vi "Run.vi"(7 "Team Index":i32, 8 "Column":i32, 9 "Row":i32, 10 "View":i32[](array[numeric]) caption="View (Team Index, -1: empty)", 11 "Team 3 In":refnum<class "Team 3.lvclass">) -> (0 "Replicated":refnum<class "Square.lvclass">, 1 "Direction":T1, 2 "Action":T2, 3 "Square Out":refnum<class "Square.lvclass">)   [LabVIEW 2020, in "Team 3.lvclass"]
uses:
  Team 3.lvclass
  C:/dev/IlluminatedG/sol-squarebattle/Square/Square.lvclass
  Square/Square.lvclass
  Type Defs/Action Enum.ctl
  Type Defs/Direction Enum.ctl
  Team 3.lvclass/Team 3.ctl
  SubVIs/Read-Only Globals.vi
  SubVIs/Globals (private).vi
  SubVIs/Read-Only Stats.vi
  DS Square Library/DS Square.lvlib
  Type Defs/SB Type Defs.lvlib
panel:
  # "NW\nN\nNE\nE\nSE\nS\nSW\nW"
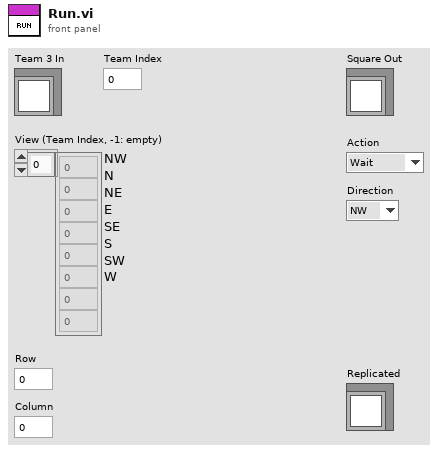
[diagram p1: front panel]
types:
  T1 = typedef "SB Type Defs.lvlib/Direction Enum.ctl" = enum16{"NW", "N", "NE", "E", "SE", "S", "SW", "W"}
  T2 = typedef "SB Type Defs.lvlib/Action Enum.ctl" = enum16{"Wait", "Move", "Attack", "Replicate"}
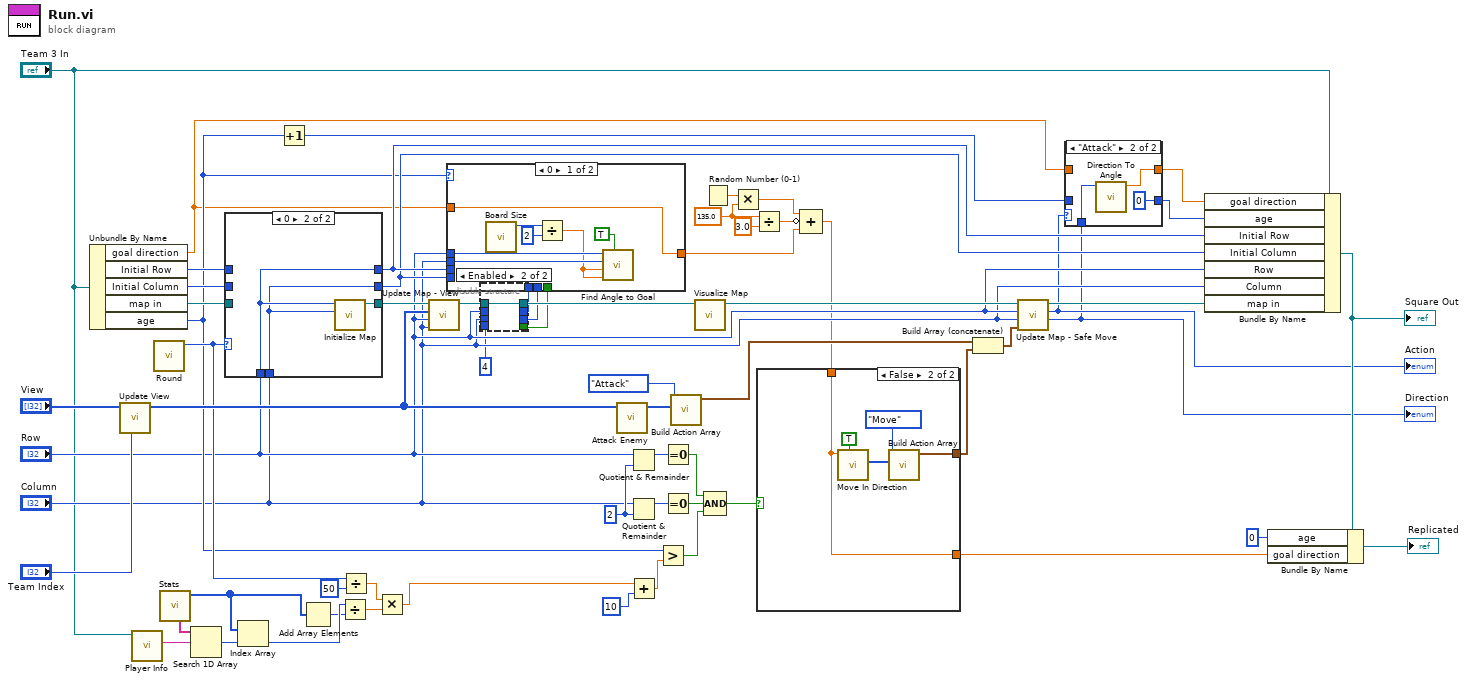
[diagram p0: block diagram]
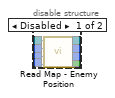
[diagram p3: hidden frame]
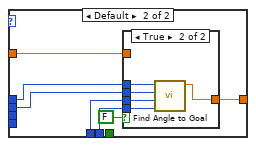
[diagram p4: hidden frame]
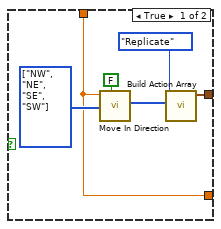
[diagram p6: hidden frame]
diagram:
  w41 = 135.0 ("y")
  w59 = 2 ("y")
  n1 = Unbundle By Name("Team 3 In") -> ("goal direction"=w1:dbl, "Initial Row"=w38:i32, "Initial Column"=w37:i32, "map in"=w63:refnum<data-value>, "age"=w28:i32)
  n2 = call "Update View.vi"("Team Index"="Team Index", "View"="View") -> ("View out"=w53:i32[])  [unwired: 9 in]
  n3 = call-dynamic "Player Info.vi"("Team 3 in"="Team 3 In") -> ("Name"=w17:string)  [unwired: 7 in, 3 out]
  n4 = call "Round.vi"() -> ("Round"=w31:i32)  [unwired: 11 in]
  n5 = call "Stats.vi"() -> ("Squares"=w16:i32[], "Players"=w18:string[])  [unwired: 7 in, 3 out]
  n6 = Search 1D Array(1D array=w18, element=w17) -> (index of element=w15:i32)  [unwired: 1 in]
  n7 = case shown="0" w31 {
    tunnel: w63 -> [w66 _]
    tunnel: [w66 w69] -> w62
    tunnel: "Column" -> [_ w67]
    tunnel: "Row" -> [_ w68]
    tunnel: w38 -> [w65 _]
    tunnel: w37 -> [w64 _]
    tunnel: [w65 w68] -> w36
    tunnel: [w64 w67] -> w35
    frame Default {
    }
    frame 0 {
      n8 = call "Initialize Map.vi"("Column"=w67, "Row"=w68) -> ("map"=w69:refnum<data-value>)  [unwired: 9 in]
    }
  }
  n9 = Index Array(array=w16, index=w15) -> (element=w14:i32)
  n10 = Increment(x=w28) -> (x+1=w4:i32)
  n11 = Add Array Elements(numeric array=w16) -> (sum=w13:i32)
  n12 = Divide(x=w14, y=w13) -> (x/y=w11:dbl)
  n13 = Divide(x=w31, y=50) -> (x/y=w12:dbl)
  n14 = Multiply(x=w12, y=w11) -> (x*y=w10:dbl)
  n15 = call "Update Map - View.vi"("Column"="Column", "Row"="Row", "Updated View"=w53, "map in"=w62) -> ("map out"=w27:refnum<data-value>)  [unwired: 7 in]
  n16 = disable-structure shown="Enabled" {
    disable-tunnel: w27 -> [w77 w78]
    disable-tunnel: [w76 w78] -> w26
    disable-tunnel: "Row" -> [w75 _]
    disable-tunnel: "Column" -> [w74 _]
    disable-tunnel: [w73 _] -> w23
    disable-tunnel: [w72 _] -> w22
    disable-tunnel: [w71 _] -> w21
    disable-tunnel: 4 ("distance (10)") -> [w70 _]
    frame Disabled {
      n17 = call "Read Map - Enemy Position.vi"("distance (10)"=w70, "column"=w74, "row"=w75, "map in"=w77) -> ("found?"=w73:bool, "enemy column"=w72:i32, "enemy row"=w71:i32, "map out"=w76:refnum<data-value>)  [unwired: 3 in, 1 out]
    }
    frame Enabled {
    }
  }
  n18 = case shown="0" w28 {
    tunnel: "Row" -> [w85 w91]
    tunnel: "Column" -> [w84 w90]
    tunnel: w36 -> [_ _]
    tunnel: w35 -> [_ _]
    tunnel: [w79 w92] -> w9
    tunnel: w1 -> [w79 w89]
    tunnel: w23 -> [_ _]
    tunnel: w22 -> [_ w88]
    tunnel: w21 -> [_ w87]
    frame 0 {
      n19 = call "Board Size.vi"() -> ("Board Size"=w82:i32)  [unwired: 11 in]
      n20 = Divide(x=w82, y=2) -> (x/y=w80:dbl)
      n21 = call "Find Angle to Goal.vi"("rollover?"=TRUE, "Goal Column"=w80, "Goal Row"=w80, "Column"=w84, "Row"=w85) -> ()  [unwired: 3 in, 4 out]
    }
    frame Default {
      n22 = case shown="True" FALSE {
        tunnel: [w93 w98] -> w92
        tunnel: w91 -> [_ w97]
        tunnel: w88 -> [_ w96]
        tunnel: w90 -> [_ w95]
        tunnel: w87 -> [_ w94]
        tunnel: w89 -> [w93 _]
        frame False {
        }
        frame True {
          n23 = call "Find Angle to Goal.vi"("Goal Column"=w96, "Goal Row"=w94, "Column"=w95, "Row"=w97) -> ("angle (deg)"=w98:dbl)  [unwired: 4 in, 3 out]
        }
      }
    }
  }
  n24 = call "Attack Enemy.vi"("View in"=w53) -> ("all enemies"=w51:T1[])  [unwired: 8 in, 2 out]
  n25 = Quotient & Remainder(x="Row", y=w59) -> (x-y*floor(x/y)=w58:i32)  [unwired: 1 out]
  n26 = Quotient & Remainder(x="Column", y=w59) -> (x-y*floor(x/y)=w57:i32)  [unwired: 1 out]
  n27 = Add(x=w10, y=10) -> (x+y=w29:dbl)
  n28 = Greater?(x=w28, y=w29) -> (0:w33:bool)
  n29 = Equal To 0?(x=w58) -> (x = 0?=w55:bool)
  n30 = Equal To 0?(x=w57) -> (x = 0?=w54:bool)
  n31 = call "Build Action Array.vi"("directions"=w51, "Action"=Action_Enum."Attack") -> ("actions"=w49:cluster{"Action":T2, "Direction":T1}[])  [unwired: 9 in]
  n32 = call "Visualize Map.vi"("map in"=w26) -> ("map out"=w43:refnum<data-value>)  [unwired: 10 in]
  n33 = Random Number (0-1)() -> (number: 0 to 1=w42:dbl)
  n34 = Compound Arithmetic op=AND(w55, w54, w33) -> (w56:bool)
  n35 = Multiply(x=w42, y=w41) -> (x*y=w40:dbl)
  n36 = Divide(x=w41, y=3.0) -> (x/y=w39:dbl)
  n37 = Compound Arithmetic op=ADD(w40, invert w39, w9) -> (w8:dbl)
  n38 = case shown="False" w56 {
    tunnel: [w103 w109] -> w52
    tunnel: [w99 w105] -> w44
    tunnel: w8 -> [w99 w105]
    frame True {
      w101 = T1[] [enum."NW", enum."NE", enum."SE", enum."SW"] items=["NW", "N", "NE", "E", "SE", "S", "SW", "W"] ("directions")
      n39 = call "Move In Direction.vi"("move toward? (T)"=FALSE, "direction options"=w101, "goal angle (deg)"=w99) -> ("ordered directions"=w100:T1[])  [unwired: 7 in, 1 out]
      n40 = call "Build Action Array.vi"("directions"=w100, "Action"=Action_Enum."Replicate") -> ("actions"=w103:cluster{"Action":T2, "Direction":T1}[])  [unwired: 9 in]
    }
    frame False {
      n41 = call "Move In Direction.vi"("move toward? (T)"=TRUE, "goal angle (deg)"=w105) -> ("ordered directions"=w106:T1[])  [unwired: 8 in, 1 out]
      n42 = call "Build Action Array.vi"("directions"=w106, "Action"=Action_Enum."Move") -> ("actions"=w109:cluster{"Action":T2, "Direction":T1}[])  [unwired: 9 in]
    }
  }
  n43 = Build Array (concatenate)(w49, w52) -> (w48:cluster{"Action":T2, "Direction":T1}[])
  n44 = call "Update Map - Safe Move.vi"("Action Order"=w48, "Column"="Column", "Row"="Row", "map in"=w43) -> ("Selected Direction"=w5:T1, "Selected Action"=w6:T2, "map out"=w47:refnum<data-value>)  [unwired: 4 in, 1 out]
  "Action" <- w6
  "Direction" <- w5
  n45 = case shown="\"Attack\"" w6 {
    tunnel: w5 -> [_ w114]
    tunnel: [w110 w113] -> w2
    tunnel: w4 -> [w111 _]
    tunnel: [w111 0] -> w3
    tunnel: w1 -> [w110 _]
    frame Default {
    }
    frame "Attack" {
      n46 = call "Direction To Angle.vi"("Direction"=w114) -> ("angle (deg)"=w113:dbl)  [unwired: 10 in]
    }
  }
  n47 = Bundle By Name(cluster="Team 3 In", "goal direction"=w2, "age"=w3, "Initial Row"=w36, "Initial Column"=w35, "Row"="Row", "Column"="Column", "map in"=w47) -> (w46:refnum<class "Team 3.lvclass">)
  "Square Out" <- w46
  n48 = Bundle By Name(cluster=w46, "age"=0, "goal direction"=w44) -> (→"Replicated":refnum<class "Team 3.lvclass">)
